vi "Apply Voltage.vi"(8 "error in (no error)":errorcluster, 11 "Tool Funnel in":refnum<class "Tool Funnel.lvclass">) -> (0 "error out":errorcluster, 3 "Tool Funnel out":refnum<class "Tool Funnel.lvclass">)   [LabVIEW 2019, in "Tool Funnel.lvclass"]
uses:
  Tool Funnel.lvclass
  Settings/ObjectSettings/ObjectSettings.lvclass/ObjectSettings.ctl
  Settings/Funnel Settings/Funnel Settings.lvclass
  C:/Users/Albro/Documents/GitHub/AFM-Lithography/lvsrc/Classes/Settings/ObjectSettings/ObjectSettings.lvclass
  Settings/ObjectSettings/ObjectSettings.lvclass
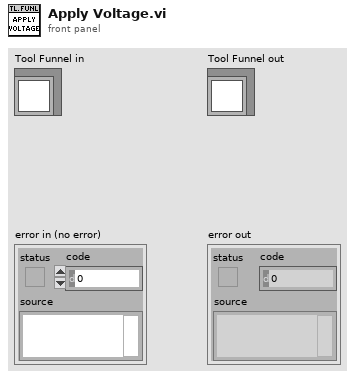
[diagram p1: front panel]
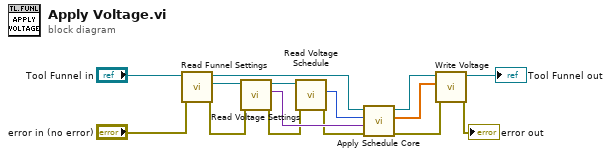
[diagram p0: block diagram]
diagram:
  n1 = call-dynamic "Read Funnel Settings.vi"("error in (no error)"="error in (no error)", "Tool Funnel in"="Tool Funnel in") -> ("error out"=w4:errorcluster, "Funnel Settings.lvclass"=w3:refnum<class "Funnel Settings.lvclass">, "Tool Funnel out"=w6:refnum<class "Tool Funnel.lvclass">)  [unwired: 7 in]
  n2 = call "Read Voltage Settings.vi"("error in (no error)"=w4, "ObjectSettings in"=w3) -> ("error out"=w9:errorcluster, "Settings"=w14:variant, "ObjectSettings out"=w15:refnum<class "Funnel Settings.lvclass">)  [unwired: 7 in]
  n3 = call "Read Voltage Schedule.vi"("error in (no error)"=w9, "ObjectSettings in"=w15) -> ("error out"=w12:errorcluster, "Schedule"=w13:u16)  [unwired: 7 in, 1 out]
  n4 = call-dynamic "Apply Schedule Core.vi"("error in (no error)"=w12, "Settings"=w14, "Schedule"=w13, "Tool Object in"=w6) -> ("error out"=w11:errorcluster, "Schedule Array"=w8:dbl[], "Tool Object out"=w10:refnum<class "Tool Funnel.lvclass">)  [unwired: 5 in]
  n5 = call-dynamic "Write Voltage.vi"("error in (no error)"=w11, "Voltage"=w8, "Tool Object in"=w10) -> ("error out"=→"error out":errorcluster, "Tool Object out"=→"Tool Funnel out":refnum<class "Tool Funnel.lvclass">)  [unwired: 7 in]
